vi "Bejelentkezés.vi"(8 "Error In":errorcluster, 10 "Message Queue":refnum<queue>, 11 "Felhasználói adatok in":string[][](array[string])) -> (0 "Error Out":errorcluster, 2 "OK ?":bool, 3 "Felhasználó ki":T2)   [LabVIEW 2014]
uses:
  support/Message Queue/Message Cluster.ctl
  <vilib>/Utility/miscctls.llb/LVRectTypeDef.ctl
  <vilib>/Utility/miscctls.llb/LVPointTypeDef.ctl
  <vilib>/event_ctls.llb/eventvkey.ctl
  support/Message Queue/Message Queue.lvlib
panel:
  in  "NumPad":T1
  out "Hibás jelszó":string
  out "Hibás név":string
  in  "Jelszó:":string
  in  "NÉV:":string(combo)
  in  "Cancel Button":bool
  in  "OK Button":bool
  # "Bejelentkezés"
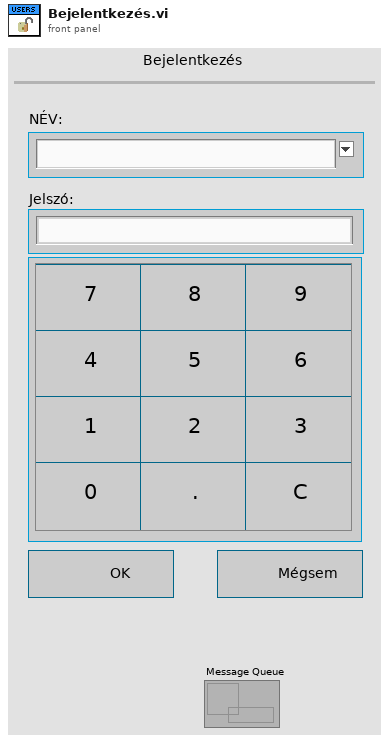
[diagram p1: front panel]
types:
  T1 = cluster{"0":bool, "1":bool, "2":bool, "3":bool, "4":bool, "5":bool, "6":bool, "7":bool, "8":bool, "9":bool, ".":bool, "C":bool}
  T2 = typedef "Felhasználó típus.ctl" = cluster{"NÉV:":string, "Jelszó: (csak számjegyek)":string, "Felhasználói szint":string}
  T3 = typedef "LVPointTypeDef.ctl" = cluster{"Horizontal":i16, "Vertical":i16}
  T4 = typedef "LVRectTypeDef.ctl" = cluster{"Left":i16, "Top":i16, "Right":i16, "Bottom":i16}
  T5 = typedef "eventvkey.ctl" = enum16{"ASCII", "Enter", "Return", "Shift", "Ctrl", "Alt", "Cmd", "Opt", "Caps", "NumLock", "Clear", "Break", "Up", "Down", "Left", "Right", "Insert", "Delete", "Home", "End", "PageUp", "PageDown", "Escape", "Help", "Pause", "ScrollLock", "F1", "F2", "F3", "F4", "F5", "F6", "F7", "F8", "F9", "F10", "F11", "F12", "F13", "F14", "F15", "F16", "F17", "F18", "F19", "F20", "F21", "F22", "F23", "F24", "Play", "VolumeUp", "VolumeDown", "Mute", "Two Byte Char"}
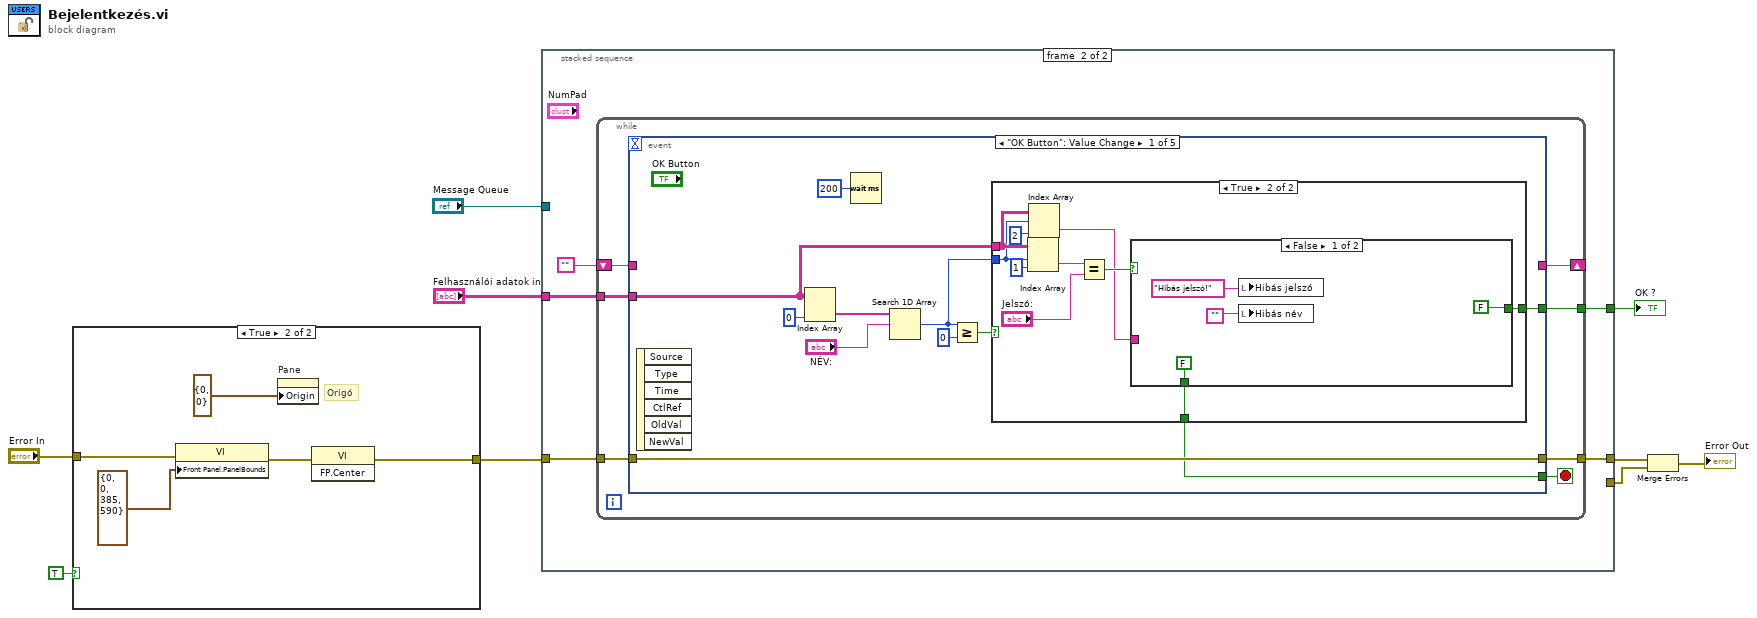
[diagram p0: block diagram]
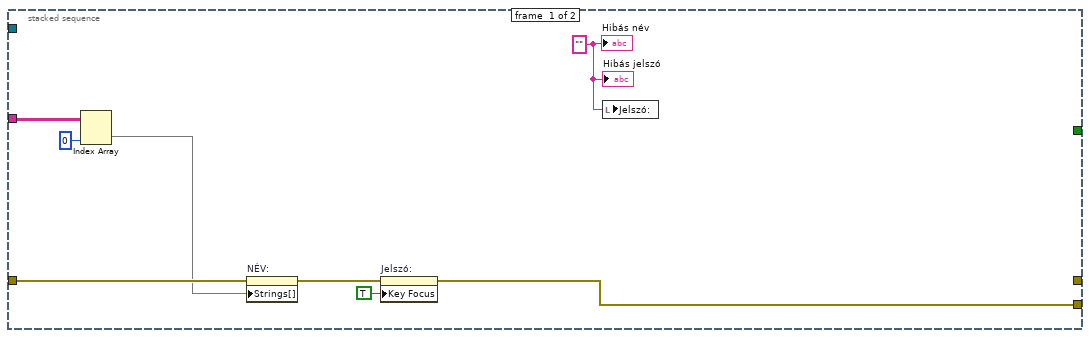
[diagram p3: hidden frame]
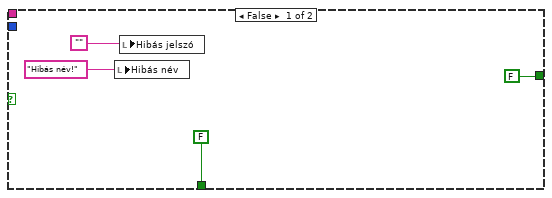
[diagram p4: hidden frame]
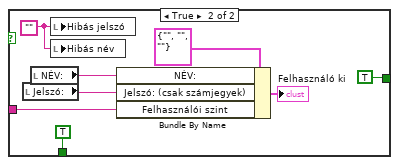
[diagram p5: hidden frame]
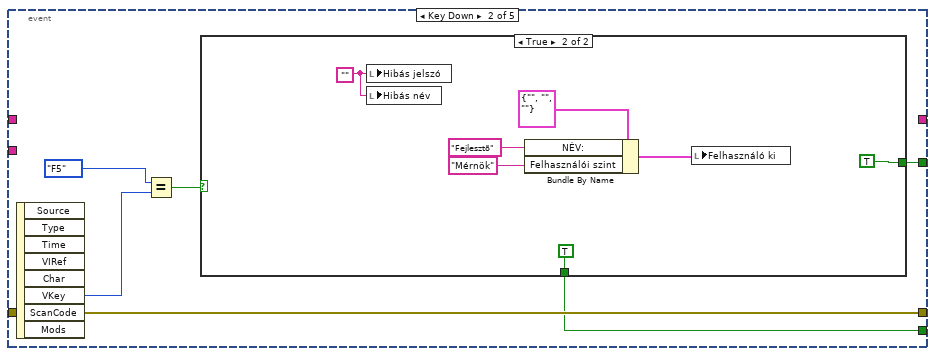
[diagram p6: hidden frame]
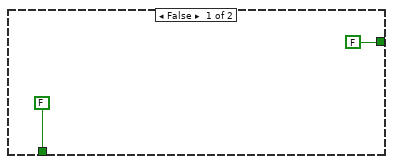
[diagram p7: hidden frame]
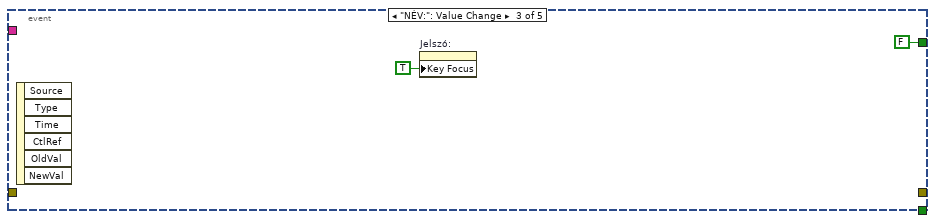
[diagram p8: hidden frame]
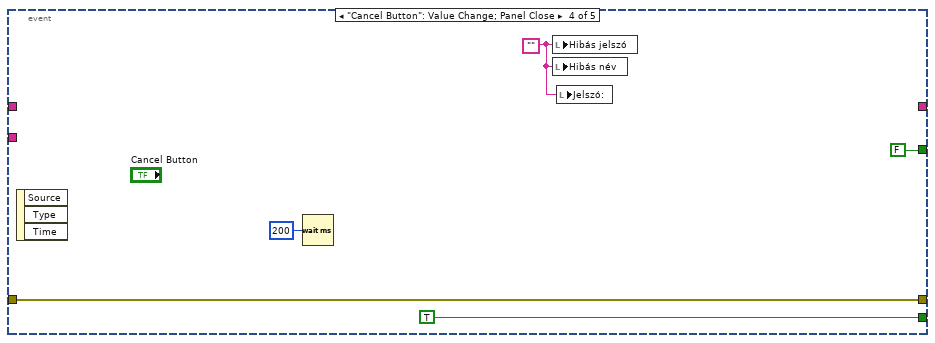
[diagram p9: hidden frame]
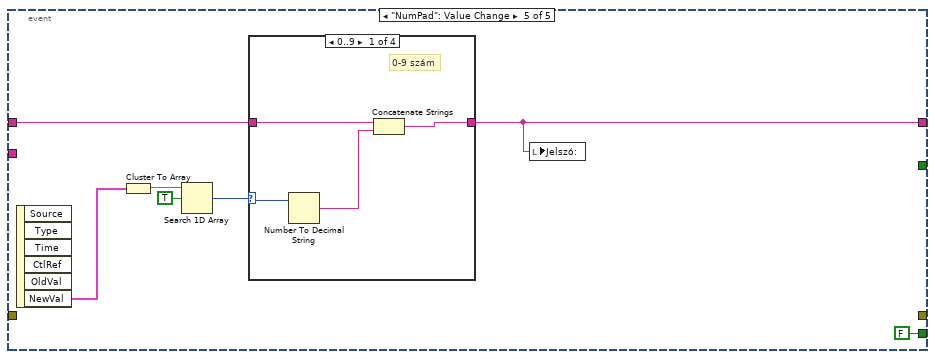
[diagram p10: hidden frame]
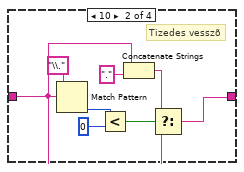
[diagram p11: hidden frame]
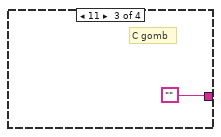
[diagram p12: hidden frame]
diagram:
  n1 = case shown="True" TRUE {
    tunnel: "Error In" -> [w10 w13]
    tunnel: [w10 w11] -> w3
    frame False {
    }
    frame True {
      # "Origó"
      n2 = property class="VI"(error in=w13, "Front Panel.PanelBounds"=T4 {"Left"=0, "Top"=0, "Right"=385, "Bottom"=590} ("Front Panel Window:Panel Bounds")) -> (error out=w12:errorcluster)  [unwired: 1 in, 1 out]
      n3 = property on="Pane" class="Pane"("Origin"=T3 {"Horizontal"=0, "Vertical"=0}) -> ()  [unwired: 2 in, 2 out]
      n4 = invoke class="VI" method="FP.Center"(error in=w12) -> (error out=w11:errorcluster)  [unwired: 2 in, 2 out]
    }
  }
  n5 = stacked-sequence {
    tunnel: w3 -> [w18 w28]
    tunnel: [_ w27] -> w7
    tunnel: "Felhasználói adatok in" -> [w19 w26]
    tunnel: [_ w25] -> w8
    tunnel: [w21 _] -> w6
    tunnel: "Message Queue" -> [_ _]
    frame #0 {
      w23 = "" ("Hibás név")
      n6 = Index Array(array=w19, index (col)=0 ("disabled index (col)")) -> (element=w16:string[])  [unwired: 1 in]
      n7 = property on="NÉV:" class="CmbBox"(error in=w18, "Strings[]"=w16) -> (error out=w17:errorcluster)  [unwired: 1 in, 1 out]
      n8 = property on="Jelszó:" class="Str"(error in=w17, "Key Focus"=TRUE) -> (error out=w21:errorcluster)  [unwired: 1 in, 1 out]
      n9 = local write "Jelszó:"(w23) -> ()
      "Hibás név" <- w23
      "Hibás jelszó" <- w23
    }
    frame #1 {
      n10 = while {
        tunnel: w28 -> [w34]
        tunnel: [w33] -> w27
        tunnel: w26 -> [w32]
        tunnel: [w31] -> w25
        shift-right: [w29] -> _
        shift-left: "" -> [w30]
        stop <- w35 stop-if-true
        n11 = event shown="[0] \"OK Button\": Value Change" {
          selector: _ -> [_ _ _ _ _]
          dyn-events: _ -> [_ _ _ _ _]
          timeout: _ -> [_ _ _ _ _]
          tunnel: [w37 w77 _ TRUE FALSE] -> w35
          tunnel: [w45 w78 _ w92 _] -> w33
          tunnel: w34 -> [w45 w78 _ w92 _]
          tunnel: w32 -> [w40 _ _ _ _]
          tunnel: [w36 w76 FALSE FALSE _] -> w31
          tunnel: w30 -> [_ _ _ _ w97]
          tunnel: [_ _ _ _ w96] -> w29
          event "OK Button": Value Change {
            n12 = event-data() -> ()  [unwired: 1 in, 6 out]
            n13 = Index Array(array=w40, index (col)=0 ("disabled index (col)")) -> (element=w43:string[])  [unwired: 1 in]
            n14 = Wait (ms)(milliseconds to wait=u32 200) -> ()  [unwired: 1 out]
            n15 = Search 1D Array(1D array=w43, element="NÉV:") -> (index of element=w39:i32)  [unwired: 1 in]
            n16 = Greater Or Equal?(x=w39, y=0) -> (x >= y?=w38:bool)
            n17 = case shown="True" w38 {
              tunnel: w40 -> [_ w55]
              tunnel: w39 -> [_ w54]
              tunnel: [FALSE w57] -> w37
              tunnel: [FALSE w51] -> w36
              frame False {
                n18 = local write "Hibás név"("Hibás név!" ("Hibás jelszó")) -> ()
                n19 = local write "Hibás jelszó"("") -> ()
              }
              frame True {
                n20 = Index Array(array=w55, index (row)=w54, index (col)=1 ("disabled index (col)")) -> (element=w59:string)
                n21 = Index Array(array=w55, index (row)=w54, index (col)=2 ("disabled index (col)")) -> (element=w52:string)
                n22 = Equal?(x=w59, y="Jelszó:") -> (x = y?=w56:bool)
                n23 = case shown="False" w56 {
                  tunnel: [FALSE TRUE] -> w57
                  tunnel: w52 -> [_ w68]
                  tunnel: [FALSE TRUE] -> w51
                  frame False {
                    n24 = local write "Hibás jelszó"("Hibás jelszó!" ("Hibás jelszó")) -> ()
                    n25 = local write "Hibás név"("") -> ()
                  }
                  frame True {
                    w71 = ""
                    n26 = local read "Jelszó:"() -> (w69:string)
                    n27 = local read "NÉV:"() -> (w70:string)
                    n28 = local write "Hibás jelszó"(w71) -> ()
                    n29 = local write "Hibás név"(w71) -> ()
                    n30 = Bundle By Name(cluster=T2 {"NÉV:"="", "Jelszó: (csak számjegyek)"="", "Felhasználói szint"=""} ("Felhasználói adatok in"), "NÉV:"=w70, "Jelszó: (csak számjegyek)"=w69, "Felhasználói szint"=w68) -> (→"Felhasználó ki":T2)
                  }
                }
              }
            }
          }
          event Key Down {
            n31 = event-data() -> ("VKey"=w74:T5)  [unwired: 1 in, 7 out]
            n32 = Equal?(x=eventvkey."F5" ("VKey"), y=w74) -> (x = y?=w75:bool)
            n33 = case shown="True" w75 {
              tunnel: [FALSE TRUE] -> w77
              tunnel: [FALSE TRUE] -> w76
              frame False {
              }
              frame True {
                w85 = ""
                n34 = local write "Hibás jelszó"(w85) -> ()
                n35 = local write "Hibás név"(w85) -> ()
                n36 = Bundle By Name(cluster=T2 {"NÉV:"="", "Jelszó: (csak számjegyek)"="", "Felhasználói szint"=""} ("Felhasználói adatok in"), "NÉV:"="Fejlesztõ" ("NÉV ki"), "Felhasználói szint"="Mérnök" ("Jogosultsági szint ki")) -> (w82:T2)
                n37 = local write "Felhasználó ki"(w82) -> ()
              }
            }
          }
          event "NÉV:": Value Change {
            n38 = event-data() -> ()  [unwired: 1 in, 6 out]
            n39 = property on="Jelszó:" class="Str"("Key Focus"=TRUE) -> ()  [unwired: 2 in, 2 out]
          }
          event "Cancel Button": Value Change; Panel Close {
            w91 = ""
            n40 = event-data() -> ()  [unwired: 1 in, 3 out]
            n41 = Wait (ms)(milliseconds to wait=u32 200) -> ()  [unwired: 1 out]
            n42 = local write "Hibás jelszó"(w91) -> ()
            n43 = local write "Hibás név"(w91) -> ()
            n44 = local write "Jelszó:"(w91) -> ()
          }
          event "NumPad": Value Change {
            n45 = event-data() -> ("NewVal"=w101:T1)  [unwired: 1 in, 5 out]
            n46 = Cluster To Array(cluster=w101) -> (array=w100:bool[])
            n47 = Search 1D Array(1D array=w100, element=TRUE) -> (index of element=w98:i32)  [unwired: 1 in]
            n48 = case shown="0..9" w98 {
              selector: w98 -> [w105 _ _ _]
              tunnel: w97 -> [w104 w107 _ w115]
              tunnel: [w102 w106 "" w115] -> w96
              frame 0..9 {
                # "0-9 szám"
                n49 = Number To Decimal String(number=w105) -> (decimal integer string=w103:string)  [unwired: 1 in]
                n50 = Concatenate Strings(w104, w103) -> (w102:string)
              }
              frame 10 {
                # "Tizedes vesszõ"
                n51 = Match Pattern(string=w107, regular expression="\\.") -> (offset past match=w108:i32)  [unwired: 1 in, 3 out]
                n52 = Less?(x=w108, y=0) -> (x < y?=w110:bool)
                n53 = Concatenate Strings(w107, "." ("regular expression")) -> (w111:string)
                n54 = Select(t=w111, s=w110, f=w107) -> (s? t:f=w106:string)
              }
              frame 11 {
                # "C gomb"
              }
              frame Default {
              }
            }
            n55 = local write "Jelszó:"(w96) -> ()
          }
        }
      }
    }
  }
  "OK ?" <- w8
  n56 = Merge Errors(w7, w6) -> (→"Error Out":errorcluster)
